vi "Arduino Photocell.vi"() -> ()   [LabVIEW 2011, in "LabVIEW Interface for Arduino.lvlib"]
doc: "An example that uses the Arduino to read the value of a photocell."
uses:
  vi.lib/LabVIEW Interface for Arduino/LabVIEW Interface for Arduino.lvlib
  vi.lib/LabVIEW Interface for Arduino/Private/Type Defs/Analog Pin.ctl
panel:
  in  "VISA resource name":refnum<visa-resource-name>
  in  "Stop":bool
  out "Light Intensity (0 - 100)":dbl(knob) scale=0.0..100.0
  in  "Photo Cell Pin (AI 0-5)":T1=enum."AI_1"
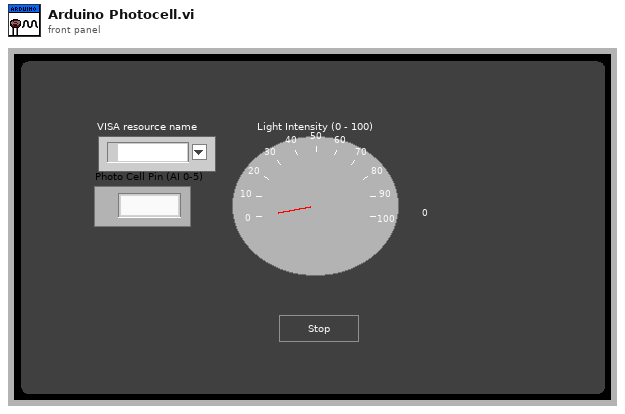
[diagram p1: front panel]
types:
  T1 = typedef "LabVIEW Interface for Arduino.lvlib/Analog Pin.ctl" = enum8{"AI_0", "AI_1", "AI_2", "AI_3", "AI_4", "AI_5", "AI_6", "AI_7", "AI_8", "AI_9", "AI_10", "AI_11", "AI_12", "AI_13", "AI_14", "AI_15"}
  T2 = typedef "LabVIEW Interface for Arduino.lvlib/Arduino Resource.ctl" = cluster{"VISA resource":refnum<visa-resource-name>, "Board Type":T3, "Connection Type":enum8{"USB / Serial"}, "Bytes Per Packet (15)":u8}
  T3 = typedef "LabVIEW Interface for Arduino.lvlib/Board Type.ctl" = enum16{"Arduino Uno", "Dimuelanove w/Atmega 328", "Mega 2560", "Chipkit Uno32", "Chipkit Max32"}
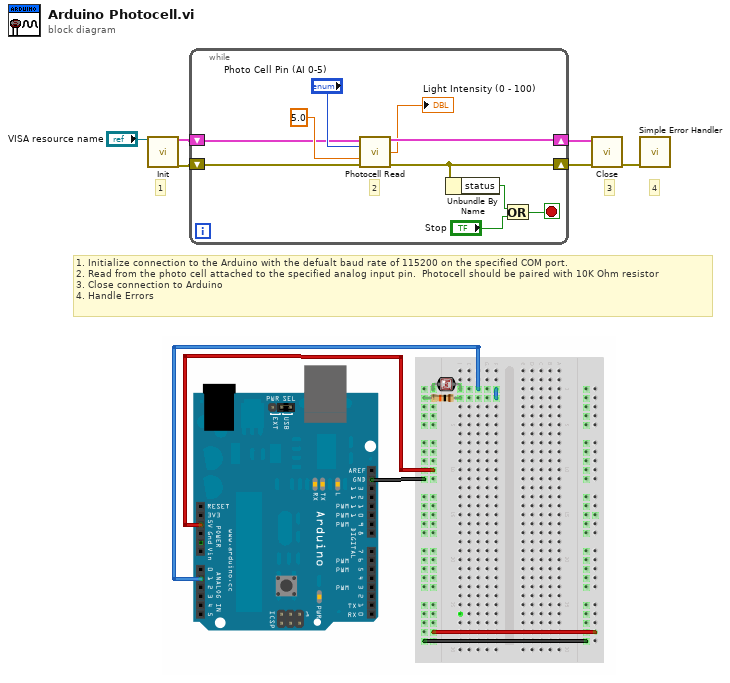
[diagram p0: block diagram]
diagram:
  # "1. Initialize connection to the Arduino with the defualt baud rate of 115200 on the specified COM port.\n2. Read from the photo cell attached to the specified analog input pin.  Photocell should be paired with 10K Ohm resistor\n3. Close connection to Arduino\n4. Handle Errors"
  # "4"
  # "3"
  # "1"
  n1 = call "Init.vi"("VISA resource"="VISA resource name") -> ("Arduino Resource"=w5:T2, "error out"=w4:errorcluster)  [unwired: 17 in]
  n2 = while {
    shift-right: [w11] -> w6
    shift-left: w4 -> [w16]
    shift-right: [w15] -> w2
    shift-left: w5 -> [w7]
    stop <- w8 stop-if-true
    # "2"
    n3 = call "Photocell Read.vi"("Arduino Resource"=w7, "Photo Cell Pin (0)"="Photo Cell Pin (AI 0-5)", "Vcc (5)"=5.0 ("Vcc"), "error in"=w16) -> ("Arduino Resource"=w15:T2, "Light Intensity (0 - 100)"=→"Light Intensity (0 - 100)":dbl, "error out"=w11:errorcluster)  [unwired: 9 in]
    n4 = Unbundle By Name(w11) -> ("status"=w10:bool)
    n5 = Or(x=w10, y="Stop") -> (x .or. y?=w8:bool)
  }
  n6 = call "Close.vi"("Arduino Resource"=w2, "error in"=w6) -> ("error out"=w3:errorcluster)  [unwired: 13 in]
  n7 = call <vilib>:"Simple Error Handler.vi"("error in (no error)"=w3) -> ()  [unwired: 4 in, 5 out]
